vi "_RT_CtrlLoop_Laser_Process.vi"(6 "ExpVar in":refnum<class "ExpVar.lvclass">, 8 "error in (no error)":errorcluster, 9 "safty":refnum<data-value>, 10 "system enable":refnum<data-value>, 11 "RS232ComPort":refnum<class "RS232ComPort.lvclass">) -> ()   [LabVIEW 2018]
uses:
  PublicSubVI/RS232/RS232ComPort.lvclass
  PublicSubVI/NewExpVar/ExpVar.lvclass
  PublicSubVI/Ctl/_ctl_RT_SysLog.ctl
  Ctl/_ctl_LaserCmd.ctl
  Ctl/_ctl_LaserParam.ctl
  Class/Laser349.lvclass
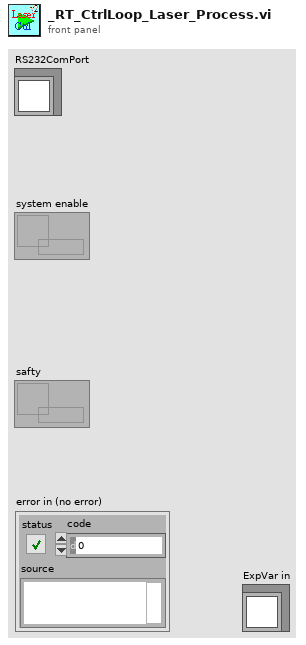
[diagram p1: front panel]
types:
  T1 = typedef "_ctl_RT_SysLog.ctl" = enum16{"None", "Initialize", "StartupRT", "StartupFPGA", "StartupAllocator", "GetMass", "SetWfmCode", "SetLaserCtrl", "SetTurboCtrl", "SetD999Ctrl", "Reconnecting...", "Interrupt", "StopRT"}
  T2 = typedef "_ctl_LaserCmd.ctl" = enum8{"Diode_On", "Diode_Off", "Standby_On", "Standby_Off", "Internal_Trig", "External_Trig", "Set_Energy", "Set_Frequency", "Read_Version", "Read_STB", "Read_Diode_TEMP", "Read_SHG_TEMP", "Read_THG_TEMP", "Read_Base_Plate_TEMP", "Read_Diode_Hour", "Read_Diode_Maxc", "Read_Diode_Curr", "Read_QSW_CNTS", "Read_PENER", "Read_Freq", "Read_PCUR", "Read_Fault_Codes"}
  T3 = typedef "_ctl_LaserParam.ctl" = cluster{"Energy":dbl, "Freq":dbl, "Emission":bool, "TriggerSource":enum16{"Internal", "External"}, "Time Stamp":timestamp}
  T4 = typedef "Semaphore RefNum" = refnum<k1>
  T5 = cluster{"Response Str":string, "VISA resource":refnum<visa-resource-name>, "DeviceExist?":bool, "semaphore":T4}
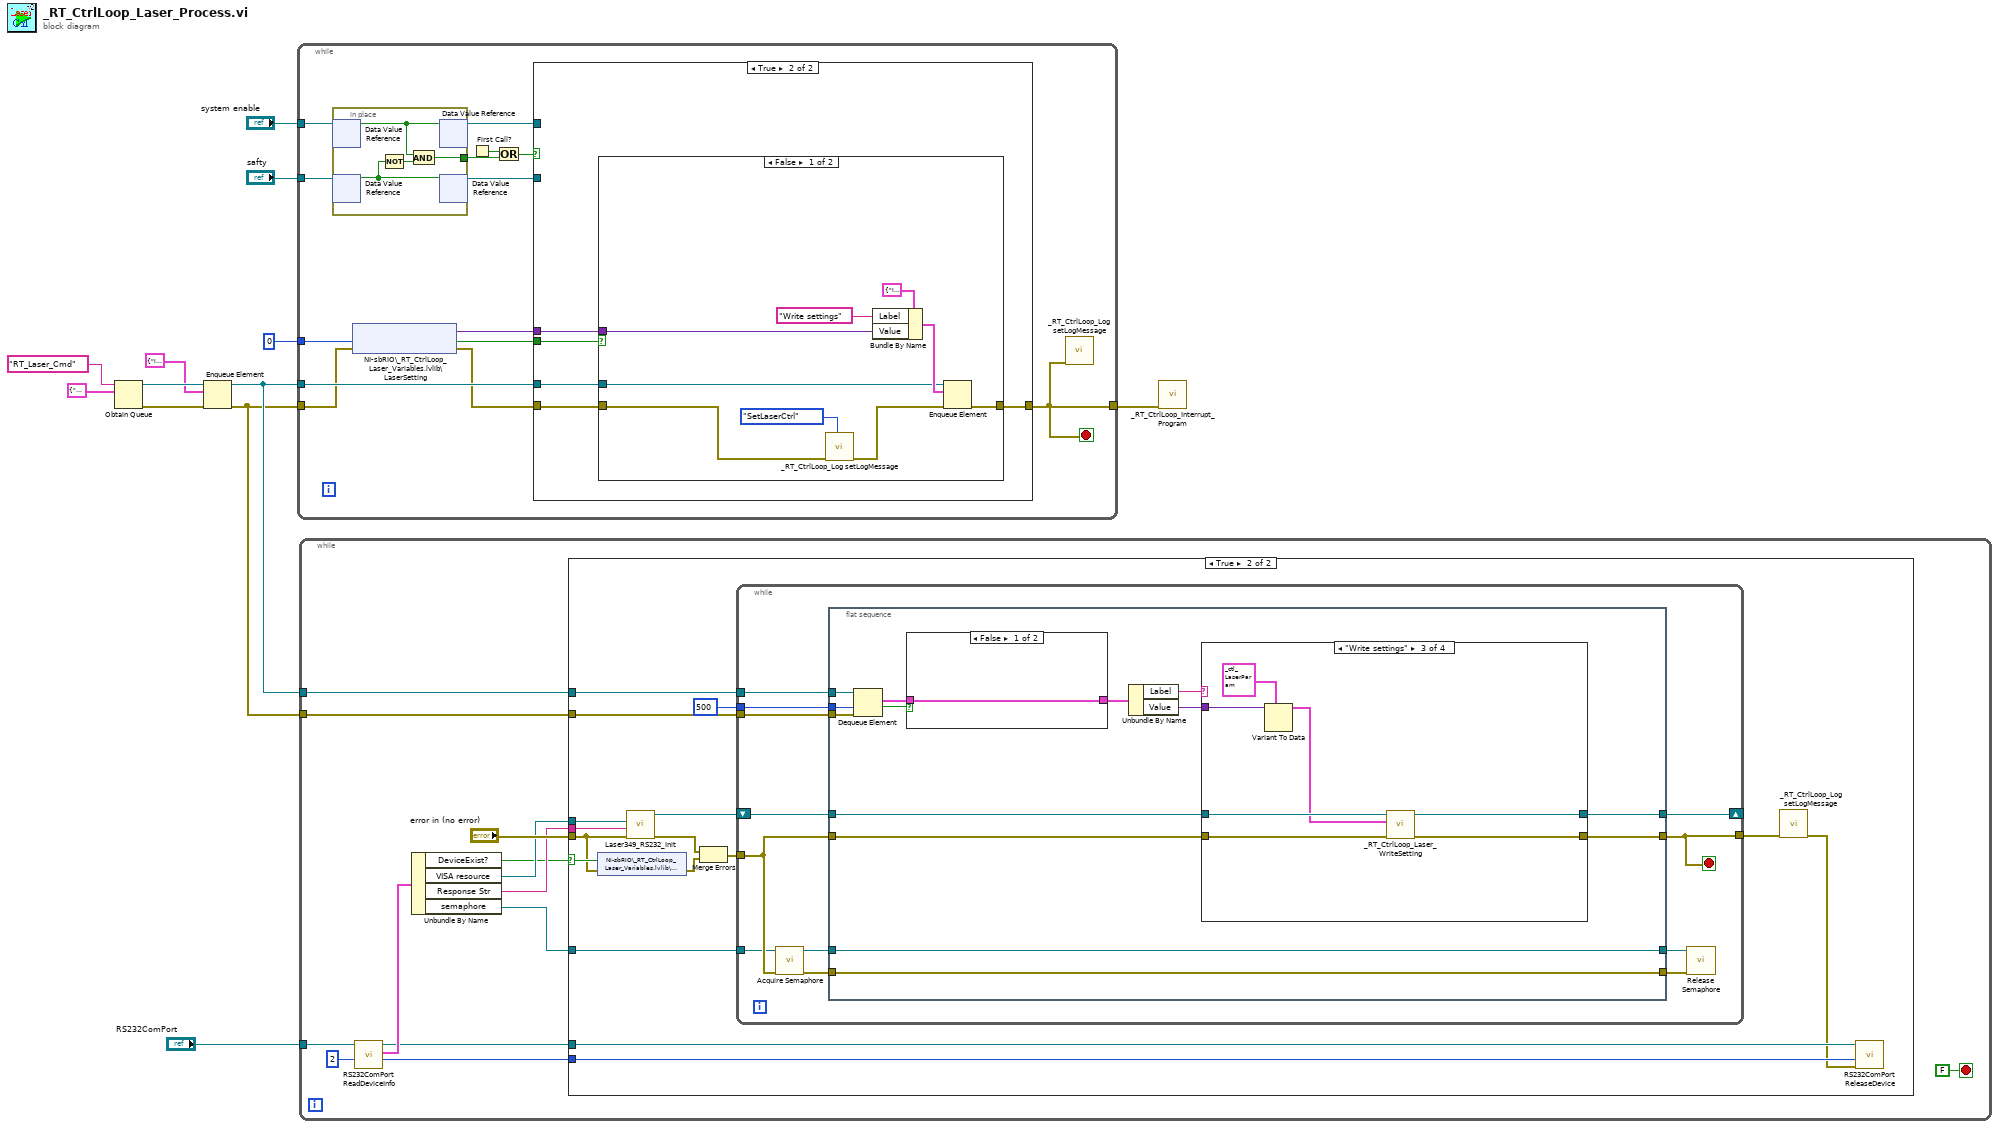
[diagram p0: block diagram]
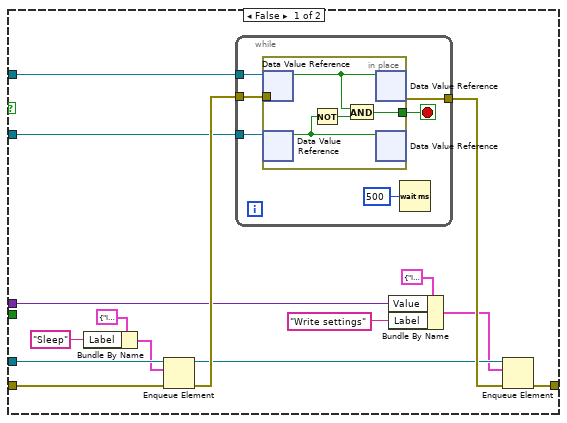
[diagram p2: hidden frame]
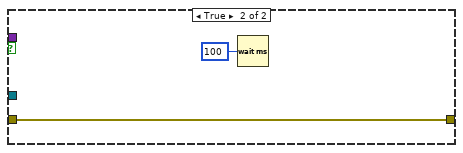
[diagram p3: hidden frame]
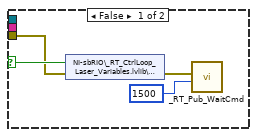
[diagram p4: hidden frame]
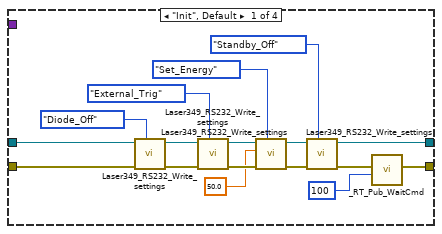
[diagram p5: hidden frame]
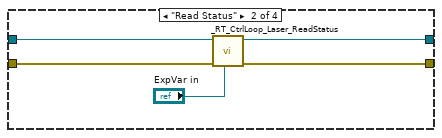
[diagram p6: hidden frame]
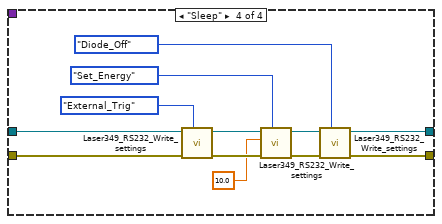
[diagram p7: hidden frame]
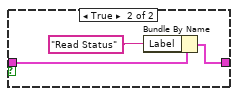
[diagram p8: hidden frame]
diagram:
  n1 = Obtain Queue(name (unnamed)="RT_Laser_Cmd", element data type=cluster{"Label":string, "Value":variant} {"Label"="", "Value"=variant}) -> (queue out=w9:refnum<queue>, error out=w8:errorcluster)  [unwired: 3 in, 1 out]
  n2 = Enqueue Element(queue=w9, element=cluster{"Label":string, "Value":variant} {"Label"="Init", "Value"=variant}, error in (no error)=w8) -> (queue out=w5:refnum<queue>, error out=w4:errorcluster)  [unwired: 1 in, 1 out]
  n3 = while {
    tunnel: w5 -> [w26]
    tunnel: w4 -> [w18]
    tunnel: 0 -> [w25]
    tunnel: "system enable" -> [w23]
    tunnel: "safty" -> [w20]
    tunnel: [w16] -> w1
    stop <- w16 stop-if-true
    n4 = in-place {
      in-place-border: [w68] -> w14
      n5 = in-place-dvr #1(w23) -> (w69:bool)  [unwired: 1 out]
      n6 = in-place-dvr #2(w20) -> (w71:bool)  [unwired: 1 out]
      n7 = Not(x=w71) -> (.not. x?=w70:bool)
      n8 = And(x=w69, y=w70) -> (x .and. y?=w68:bool)
      n9 = in-place-dvr #1(w69) -> (w22:refnum<data-value>)  [unwired: 1 out]
      n10 = in-place-dvr #2(w71) -> (w19:refnum<data-value>)  [unwired: 1 out]
    }
    n11 = shared-variable "NI-sbRIO\\_RT_CtrlLoop_Laser_Variables.lvlib\\LaserSetting"(error in=w18, w25) -> (w24:variant, error out=w17:errorcluster, w21:bool)
    n12 = First Call?() -> (First Call?: T/F=w15:bool)
    n13 = Or(x=w15, y=w14) -> (x .or. y?=w13:bool)
    n14 = case shown="True" w13 {
      tunnel: w22 -> [w41 _]
      tunnel: w26 -> [w40 w55]
      tunnel: w17 -> [w39 w54]
      tunnel: w24 -> [w31 w53]
      tunnel: w21 -> [_ w56]
      tunnel: [w28 w52] -> w16
      tunnel: w19 -> [w27 _]
      frame False {
        n15 = Bundle By Name(cluster=cluster{"Label":string, "Value":variant} {"Label"="Init", "Value"=variant} ("element"), "Label"="Sleep") -> (w36:cluster{"Label":string, "Value":variant})
        n16 = Enqueue Element(queue=w40, element=w36, error in (no error)=w39) -> (queue out=w33:refnum<queue>, error out=w35:errorcluster)  [unwired: 1 in, 1 out]
        n17 = while {
          tunnel: w41 -> [w47]
          tunnel: [w45] -> w34
          tunnel: w35 -> [w44]
          tunnel: w27 -> [w42]
          stop <- w46 stop-if-true
          n18 = in-place {
            in-place-border: [w48] -> w46
            in-place-border: w44 -> [_]
            n19 = in-place-dvr #3(w47) -> (w49:bool)  [unwired: 1 out]
            n20 = in-place-dvr #4(w42) -> (w51:bool)  [unwired: 1 out]
            n21 = Not(x=w51) -> (.not. x?=w50:bool)
            n22 = And(x=w49, y=w50) -> (x .and. y?=w48:bool)
            n23 = in-place-dvr #3(w49) -> (w45:errorcluster)  [unwired: 1 out]
            n24 = in-place-dvr #4(w51) -> ()  [unwired: 2 out]
          }
          n25 = Wait (ms)(milliseconds to wait=u32 500) -> ()  [unwired: 1 out]
        }
        n26 = Bundle By Name(cluster=cluster{"Label":string, "Value":variant} {"Label"="Init", "Value"=variant} ("element"), "Value"=w31, "Label"="Write settings") -> (w29:cluster{"Label":string, "Value":variant})
        n27 = Enqueue Element(queue=w33, element=w29, error in (no error)=w34) -> (error out=w28:errorcluster)  [unwired: 1 in, 2 out]
      }
      frame True {
        n28 = case shown="False" w56 {
          tunnel: w55 -> [w62 _]
          tunnel: w54 -> [w59 w67]
          tunnel: w53 -> [w61 _]
          tunnel: [w60 w67] -> w52
          frame False {
            n29 = call "_RT_CtrlLoop_Log setLogMessage.vi"("system type"=_ctl_RT_SysLog."SetLaserCtrl", "error in"=w59) -> ("error out"=w58:errorcluster)  [unwired: 8 in, 1 out]
            n30 = Bundle By Name(cluster=cluster{"Label":string, "Value":variant} {"Label"="Init", "Value"=variant} ("element"), "Label"="Write settings", "Value"=w61) -> (w64:cluster{"Label":string, "Value":variant})
            n31 = Enqueue Element(queue=w62, element=w64, error in (no error)=w58) -> (error out=w60:errorcluster)  [unwired: 1 in, 2 out]
          }
          frame True {
            n32 = Wait (ms)(milliseconds to wait=u32 100) -> ()  [unwired: 1 out]
          }
        }
      }
    }
    n33 = call "_RT_CtrlLoop_Log setLogMessage.vi"("error in"=w16) -> ()  [unwired: 9 in, 2 out]
  }
  n34 = while {
    tunnel: "RS232ComPort" -> [w78]
    tunnel: w5 -> [w74]
    tunnel: w4 -> [w73]
    stop <- FALSE stop-if-true
    w75 = 2 ("DeviceIndex")
    n35 = call-dynamic "RS232ComPort ReadDeviceInfo.vi"("DeviceIndex"=w75, "RS232ComPort in"=w78) -> ("DeviceInfo"=w77:T5, "RS232ComPort out"=w76:refnum<class "RS232ComPort.lvclass">)  [unwired: 7 in, 1 out]
    n36 = Unbundle By Name(w77) -> ("DeviceExist?"=w80:bool, "VISA resource"=w82:refnum<visa-resource-name>, "Response Str"=w81:string, "semaphore"=w72:T4)
    n37 = case shown="True" w80 {
      selector: w80 -> [w87 w94]
      tunnel: "error in (no error)" -> [w86 w93]
      tunnel: w82 -> [_ w103]
      tunnel: w81 -> [_ w102]
      tunnel: w76 -> [_ w100]
      tunnel: w75 -> [_ w99]
      tunnel: w74 -> [_ w98]
      tunnel: w73 -> [_ w97]
      tunnel: w72 -> [_ w95]
      frame False {
        n38 = shared-variable "NI-sbRIO\\_RT_CtrlLoop_Laser_Variables.lvlib\\LaserExist"(w87, error in=w86) -> (error out=w85:errorcluster)
        n39 = call "_RT_Pub_WaitCmd.vi"("milliseconds to wait"=u32 1500, "error in (no error)"=w85) -> ()  [unwired: 9 in, 1 out]
      }
      frame True {
        n40 = shared-variable "NI-sbRIO\\_RT_CtrlLoop_Laser_Variables.lvlib\\LaserExist"(w94, error in=w93) -> (error out=w92:errorcluster)
        n41 = call "Laser349_RS232_Init.vi"("error in (no error)"=w93, "Laser ID Str"=w102, "VISA resource name"=w103) -> ("error out"=w91:errorcluster, "Laser349 out"=w101:refnum<class "Laser349.lvclass">)  [unwired: 7 in]
        n42 = Merge Errors(w91, w92) -> (w90:errorcluster)
        n43 = while {
          tunnel: w90 -> [w108]
          shift-right: [w114] -> _
          shift-left: w101 -> [w115]
          tunnel: [w110] -> w89
          tunnel: w98 -> [w113]
          tunnel: w97 -> [w112]
          tunnel: 500 -> [w111]
          tunnel: w95 -> [w104]
          stop <- w110 stop-if-true
          n44 = call <vilib>:"Acquire Semaphore.vi"("error in (no error)"=w108, "semaphore"=w104) -> ("error out"=w107:errorcluster, "semaphore out"=w109:T4)  [unwired: 3 in, 1 out]
          n45 = flat-sequence {
            tunnel: w108 -> [w129]
            tunnel: w115 -> [w128]
            tunnel: [w127] -> w114
            tunnel: w113 -> [w126]
            tunnel: w112 -> [w125]
            tunnel: w111 -> [w124]
            tunnel: [w116] -> w110
            tunnel: w109 -> [w118]
            tunnel: w107 -> [w117]
            tunnel: [w118] -> w105
            tunnel: [w117] -> w106
            frame #0 {
              n46 = Dequeue Element(queue=w126, timeout in ms (-1)=w124, error in (no error)=w125) -> (element=w123:cluster{"Label":string, "Value":variant}, timed out?=w122:bool)  [unwired: 2 out]
              n47 = case shown="False" w122 {
                tunnel: w123 -> [w171 w174]
                tunnel: [w171 w173] -> w121
                frame False {
                }
                frame True {
                  n48 = Bundle By Name(cluster=w174, "Label"="Read Status") -> (w173:cluster{"Label":string, "Value":variant})
                }
              }
              n49 = Unbundle By Name(w121) -> ("Label"=w120:string, "Value"=w119:variant)
              n50 = case shown="\"Write settings\"" w120 {
                tunnel: [w146 w147 w157 w170] -> w127
                tunnel: [w135 w148 w152 w168] -> w116
                tunnel: w129 -> [w131 w149 w153 w164]
                tunnel: w128 -> [w134 w150 w158 w165]
                tunnel: w119 -> [_ _ w156 _]
                frame "Init", Default {
                  n51 = call-dynamic "Laser349_RS232_Write_settings.vi"("Command Status"=_ctl_LaserCmd."Diode_Off", "error in (no error)"=w131, "Laser349 in"=w134) -> ("error out"=w145:errorcluster, "Laser349 out"=w144:refnum<class "Laser349.lvclass">)  [unwired: 7 in]
                  n52 = call-dynamic "Laser349_RS232_Write_settings.vi"("Command Status"=_ctl_LaserCmd."External_Trig", "error in (no error)"=w145, "Laser349 in"=w144) -> ("error out"=w142:errorcluster, "Laser349 out"=w143:refnum<class "Laser349.lvclass">)  [unwired: 7 in]
                  n53 = call-dynamic "Laser349_RS232_Write_settings.vi"("Command Status"=_ctl_LaserCmd."Set_Energy", "error in (no error)"=w142, "Input value"=50.0, "Laser349 in"=w143) -> ("error out"=w132:errorcluster, "Laser349 out"=w133:refnum<class "Laser349.lvclass">)  [unwired: 6 in]
                  n54 = call-dynamic "Laser349_RS232_Write_settings.vi"("Command Status"=_ctl_LaserCmd."Standby_Off", "error in (no error)"=w132, "Laser349 in"=w133) -> ("error out"=w130:errorcluster, "Laser349 out"=w146:refnum<class "Laser349.lvclass">)  [unwired: 7 in]
                  n55 = call "_RT_Pub_WaitCmd.vi"("milliseconds to wait"=u32 100, "error in (no error)"=w130) -> ("error out"=w135:errorcluster)  [unwired: 9 in]
                }
                frame "Read Status" {
                  n56 = call "_RT_CtrlLoop_Laser_ReadStatus.vi"("ExpVar in"="ExpVar in", "error in (no error)"=w149, "Laser349 in"=w150) -> ("error out"=w148:errorcluster, "Laser349 out"=w147:refnum<class "Laser349.lvclass">)  [unwired: 7 in]
                }
                frame "Write settings" {
                  n57 = Variant To Data(type=T3 {"Energy"=50.0, "Freq"=100.0, "Emission"=FALSE, "TriggerSource"=enum."Internal", "Time Stamp"=timestamp(0 s since 1904-01-01)} ("input cluster"), Variant=w156) -> (data=w154:T3)  [unwired: 1 in, 1 out]
                  n58 = call "_RT_CtrlLoop_Laser_WriteSetting.vi"("error in (no error)"=w153, "input cluster"=w154, "Laser349 in"=w158) -> ("error out"=w152:errorcluster, "Laser349 out"=w157:refnum<class "Laser349.lvclass">)  [unwired: 7 in]
                }
                frame "Sleep" {
                  n59 = call-dynamic "Laser349_RS232_Write_settings.vi"("Command Status"=_ctl_LaserCmd."External_Trig", "error in (no error)"=w164, "Laser349 in"=w165) -> ("error out"=w163:errorcluster, "Laser349 out"=w166:refnum<class "Laser349.lvclass">)  [unwired: 7 in]
                  n60 = call-dynamic "Laser349_RS232_Write_settings.vi"("Command Status"=_ctl_LaserCmd."Set_Energy", "error in (no error)"=w163, "Input value"=10.0, "Laser349 in"=w166) -> ("error out"=w162:errorcluster, "Laser349 out"=w167:refnum<class "Laser349.lvclass">)  [unwired: 6 in]
                  n61 = call-dynamic "Laser349_RS232_Write_settings.vi"("Command Status"=_ctl_LaserCmd."Diode_Off", "error in (no error)"=w162, "Laser349 in"=w167) -> ("error out"=w168:errorcluster, "Laser349 out"=w170:refnum<class "Laser349.lvclass">)  [unwired: 7 in]
                }
              }
            }
          }
          n62 = call <vilib>:"Release Semaphore.vi"("error in (no error)"=w106, "semaphore"=w105) -> ()  [unwired: 4 in, 2 out]
        }
        n63 = call "_RT_CtrlLoop_Log setLogMessage.vi"("error in"=w89) -> ("error out"=w88:errorcluster)  [unwired: 9 in, 1 out]
        n64 = call "RS232ComPort ReleaseDevice.vi"("error in (no error)"=w88, "DeviceIndex"=w99, "RS232ComPort in"=w100) -> ()  [unwired: 8 in, 1 out]
      }
    }
  }
  n65 = call "_RT_CtrlLoop_Interrupt_Program.vi"("error in (no error)"=w1) -> ()  [unwired: 10 in, 1 out]
